vi "lines_per_z_step_stuff.vi"(1 "lines per z step":u16, 2 "line counter for z steps":u16, 3 ">end of line?>":bool) -> (0 "number out":u16)   [LabVIEW 2010]
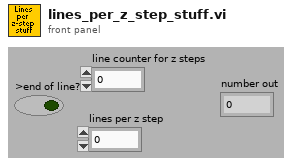
[diagram p1: front panel]
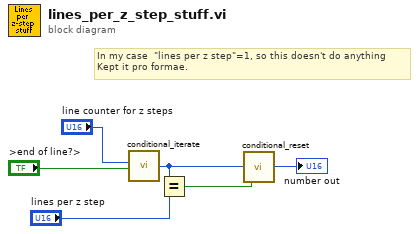
[diagram p0: block diagram]
diagram:
  # "In my case  \"lines per z step\"=1, so this doesn't do anything\nKept it pro formae."
  n1 = call "conditional_iterate.vi"("iterate?"=">end of line?>", "number in"="line counter for z steps") -> ("number out"=w3:u16)  [unwired: 4 in]
  n2 = Equal?(x=w3, y="lines per z step") -> (x = y?=w2:bool)
  n3 = call "conditional_reset.vi"("reset?"=w2, "number in"=w3) -> ("number out"=→"number out":u16)  [unwired: 4 in]
